vi "Apply System Image.vi"() -> ()   [LabVIEW 2020]
uses:
  Users/josferna/OneDrive - NI/Documents/Accounts&Proojects/Open Case Files/01072359 - Microsoft/rad-master/subVIs/Targets/TypeDefs/rad_Target Network Settings.ctl
  <vilib>/nisyscfg/Software 1.2.ctl
  <vilib>/nisyscfg/Component Type.ctl
  <vilib>/nisyscfg/Network Settings Format.ctl
  <vilib>/nisyscfg/Format With Base System Image.vi
  <vilib>/nisyscfg/Close (System).vi
  <vilib>/nisyscfg/nisyscfg.lvlib
panel:
  in  "Base System Image":T1={"title"="Linux RT System Image 20.6", "description"="", "ID"="{3CDECBF0-04E7-462E-BDD2-2AD4D9B02235}", "version"="20.6.0", "component type"=2} caption="software" {"component type" items=["standard", "hidden", "system", "unknown", "startup", "image", "essential"]}
  in  "error in":errorcluster caption="error in (no error)"
  out "error out":errorcluster
  in  "Target information":T4={"Hostname"="", "Serial number"="", "Product name"="", "Product code"=0, "System status"="", "Credential type"=enum."None/Unlocked", "User added?"=FALSE, "Primary NIC"={"MAC address"="", "IP Address Request Mode"=2, "IP address"="", "Subnet mask"="", "Gateway"="", "DNS server"=""}} {"Primary NIC"."IP Address Request Mode" items=["Static"=1, "DHCP/Link-Local"=2, "Link-Local Only"=4, "DHCP Only"=8]}
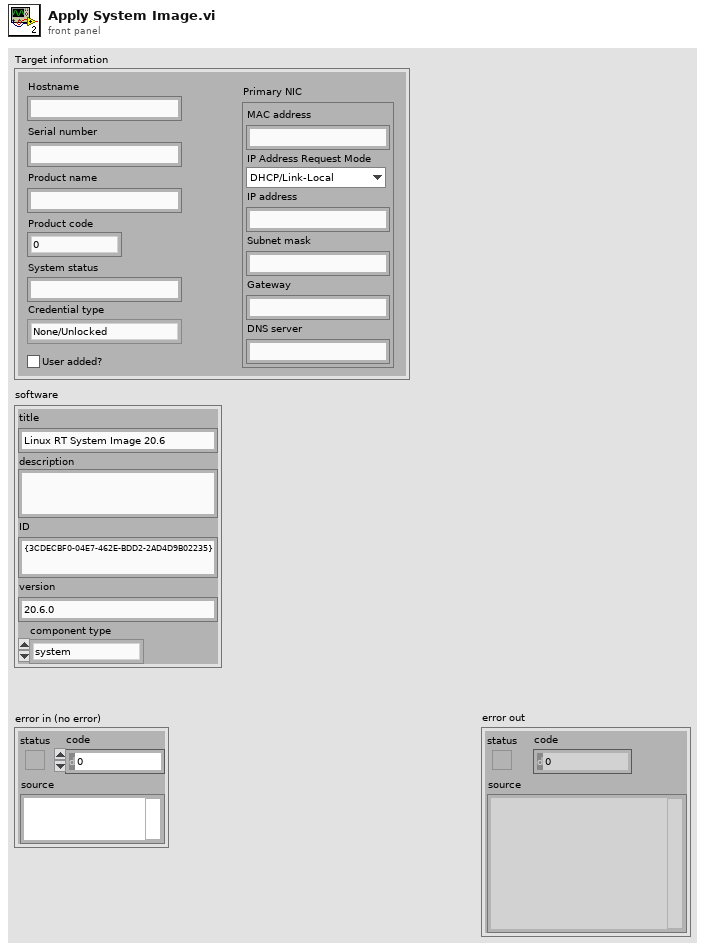
[diagram p1: front panel]
types:
  T1 = typedef "nisyscfg.lvlib/Software 1.2.ctl" = cluster{"title":string, "description":string, "ID":string, "version":string, "component type":T2}
  T2 = typedef "nisyscfg.lvlib/Component Type.ctl" = u32
  T3 = typedef "rad_Target Network Settings.ctl" = cluster{"MAC address":string, "IP Address Request Mode":i32, "IP address":string, "Subnet mask":string, "Gateway":string, "DNS server":string}
  T4 = cluster{"Hostname":string, "Serial number":string, "Product name":string, "Product code":i32, "System status":string, "Credential type":enum16{"None/Unlocked", "FTP Password", "NIAuth Credentials"}, "User added?":bool, "Primary NIC":T3}
  T5 = typedef "nisyscfg.lvlib/Network Settings Format.ctl" = u32
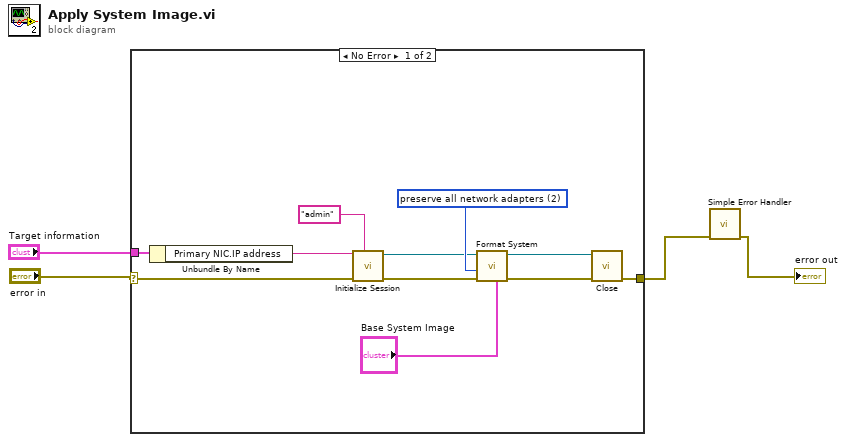
[diagram p0: block diagram]
diagram:
  n1 = case shown="No Error" "error in" {
    selector: "error in" -> [w11 w16]
    tunnel: [w15 w16] -> w2
    tunnel: "Target information" -> [w13 _]
    frame No Error {
      w10 = T5 2 items=["reset all network adapters", "preserve primary, reset others", "preserve all network adapters"] ("Network Settings (reset all adapters)")
      n2 = Unbundle By Name(w13) -> ("Primary NIC.IP address"=w12:string)
      n3 = call <vilib>:"Initialize Session.vi"("User Name"="admin", "error in (no error)"=w11, "Target (localhost)"=w12) -> ("error out"=w7:errorcluster, "Session out"=w8:refnum<k21>)  [unwired: 7 in]
      n4 = call-poly <vilib>:"Format System.vi"("Base System Image"="Base System Image", "error in (no error)"=w7, "Network Settings (reset all adapters)"=w10, "Session in"=w8) -> ("error out"=w6:errorcluster, "Session out"=w5:refnum<k21>)  [unwired: 6 in]
      n5 = call-poly <vilib>:"Close.vi"("error in (no error)"=w6, "Session in"=w5) -> ("error out"=w15:errorcluster)  [unwired: 9 in]
    }
    frame Error {
    }
  }
  n6 = call <vilib>:"Simple Error Handler.vi"("error in (no error)"=w2) -> ("error out"=→"error out":errorcluster)  [unwired: 4 in, 4 out]
